vi "SENS_IF_GAIN_LEV.vi"(0 "VISA IN":refnum<visa-resource-name>, 1 "ID":string(combo)="R1", 2 "Gain Level":enum16{"0", "1", "2"}(ring), 5 "error in":errorcluster, 7 "Channel":i32) -> (14 "VISA Out":refnum<visa-resource-name>, 19 "error out":errorcluster)   [LabVIEW 2018, in "PNA-X.lvlib"]
doc: "SENSe<cnum>:IF:GAIN:LEVel <id>, <level> \n1750\n\n(Read Write) Manually sets the gain level for the specified receiver. \nParameters \n<cnum> Existing channel number to manipulate. If unspecified, <cnum> is set to 1. \n<id> Choose from: 'A', 'B', 'R1', 'R2'. \nNote: The A and R1 receivers are always switched together. B and R2 are also \nalways switched together. For example, if you specify 'A', R1 will also be \nswitched. \n<level> Gain level. Choose from: \n0 - Lowest gain setting \n1\n2 - Highest gain setting \nExamples SENS:IF:GAIN:LEVel 'A', 1 \nQuery Syntax SENSe<cnum>:IF:GAIN:LEVel? <id> \nReturn Type Numeric \nDefault 0"
uses:
  PNA-X.lvlib
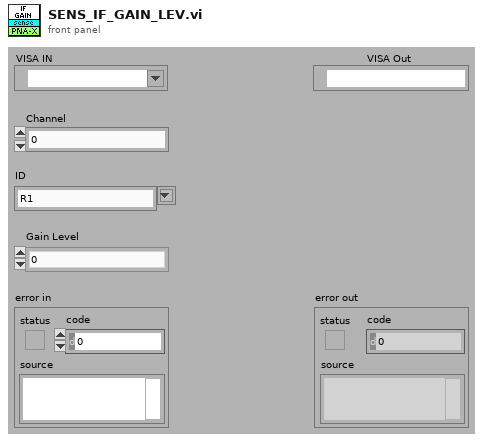
[diagram p1: front panel]
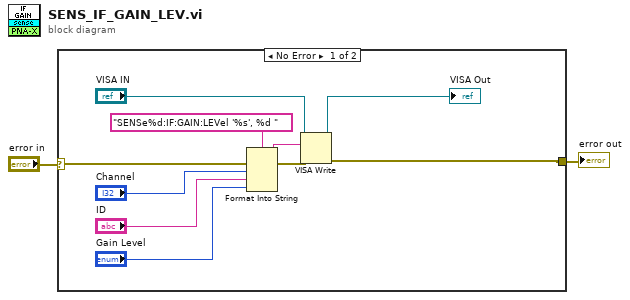
[diagram p0: block diagram]
diagram:
  n1 = case shown="No Error" "error in" {
    selector: "error in" -> [w12 w13]
    tunnel: [w7 w13] -> w1
    frame No Error {
      n2 = Format Into String(format string="SENSe%d:IF:GAIN:LEVel '%s', %d " ("Cmdline"), error in=w12, "Channel", "ID", "Gain Level") -> (resulting string=w10:string, error out=w11:errorcluster)  [unwired: 1 in]
      n3 = VISA Write(VISA resource name="VISA IN", write buffer=w10, error in (no error)=w11) -> (VISA resource name out=→"VISA Out":refnum<visa-resource-name>, error out=w7:errorcluster)  [unwired: 1 out]
    }
    frame Error {
    }
  }
  "error out" <- w1
